vi "RemoveControl.vi"(7 "Ctrl in":u32, 8 "error in":errorcluster, 9 "delay in":u32, 10 "Attrs array in":T1[](array[typedef]), 11 "Ctrl array in":u32[](array[numeric])) -> (0 "error out":errorcluster, 1 "delay out":u32, 2 "Attrs array out":T1[](array[typedef]), 3 "Ctrl array out":u32[](array[numeric]), 4 "stop?":bool)   [LabVIEW 2012, in "Spinner.xctl"]
uses:
  Spinner.xctl
  Attrs.ctl
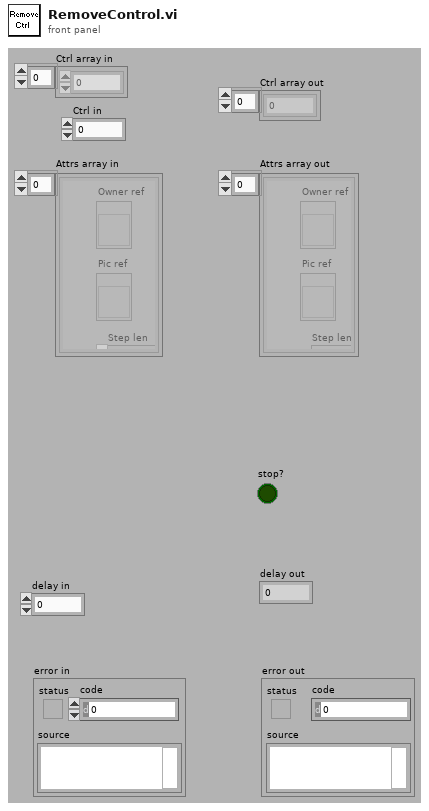
[diagram p1: front panel]
types:
  T1 = typedef "Spinner.xctl/Attrs.ctl" = cluster{"Owner ref":refnum<vi>, "Pic ref":refnum<vi>, "Step len":dbl, "Imgs":picture[], "Current phase":dbl}
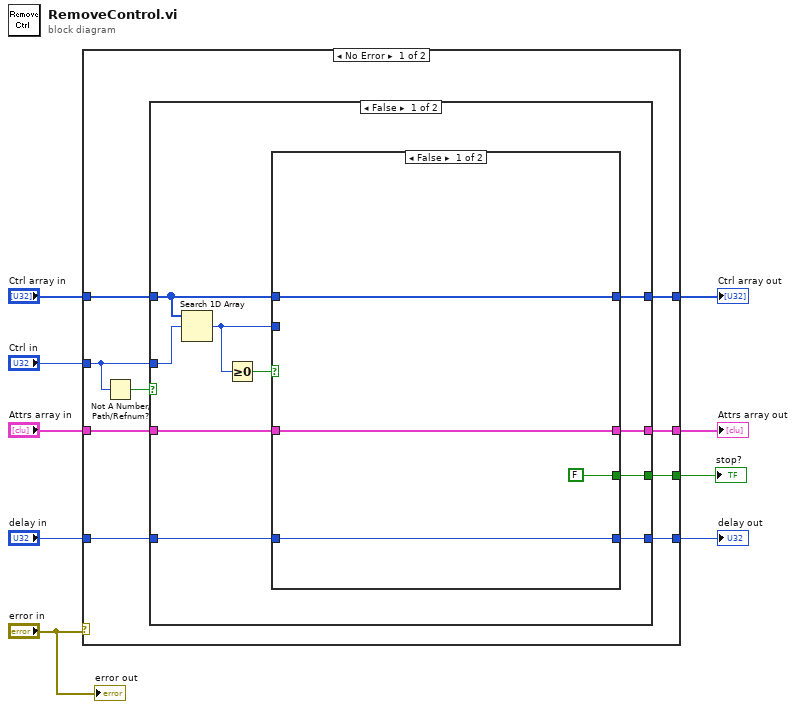
[diagram p0: block diagram]
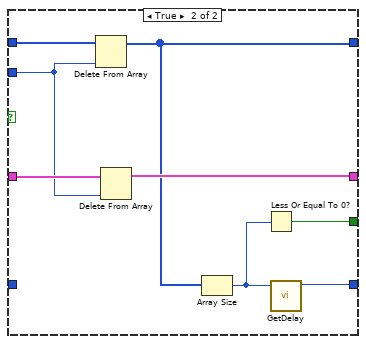
[diagram p2: hidden frame]
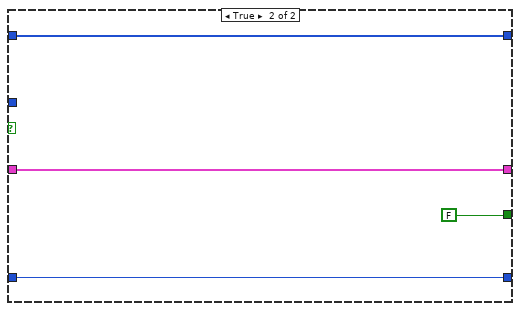
[diagram p3: hidden frame]
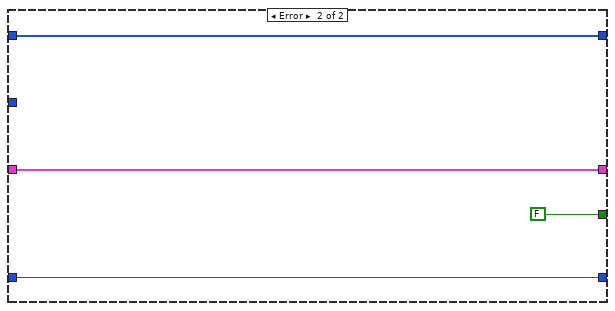
[diagram p4: hidden frame]
diagram:
  n1 = case shown="No Error" "error in" {
    tunnel: "Ctrl in" -> [w16 _]
    tunnel: "Ctrl array in" -> [w17 w48]
    tunnel: "Attrs array in" -> [w15 w47]
    tunnel: [w14 w47] -> w6
    tunnel: [w13 w48] -> w5
    tunnel: [w12 w46] -> w4
    tunnel: "delay in" -> [w11 w46]
    tunnel: [w10 FALSE] -> w1
    frame No Error {
      n2 = Not A Number/Path/Refnum?(number/path/refnum=w16) -> (NaN/Path/Refnum?=w18:bool)
      n3 = case shown="False" w18 {
        tunnel: w17 -> [w25 w44]
        tunnel: w16 -> [w24 _]
        tunnel: w15 -> [w27 w43]
        tunnel: [w26 w43] -> w14
        tunnel: [w23 w44] -> w13
        tunnel: [w22 w42] -> w12
        tunnel: w11 -> [w21 w42]
        tunnel: [w19 FALSE] -> w10
        frame False {
          n4 = Search 1D Array(1D array=w25, element=w24) -> (index of element=w20:i32)  [unwired: 1 in]
          n5 = Greater Or Equal To 0?(x=w20) -> (x >= 0?=w28:bool)
          n6 = case shown="False" w28 {
            tunnel: w27 -> [w31 w39]
            tunnel: [w31 w37] -> w26
            tunnel: w25 -> [w32 w40]
            tunnel: [w32 w35] -> w23
            tunnel: [w30 w36] -> w22
            tunnel: w21 -> [w30 _]
            tunnel: w20 -> [_ w38]
            tunnel: [FALSE w33] -> w19
            frame False {
            }
            frame True {
              n7 = Delete From Array(array=w40, index=w38) -> (array with subset deleted=w35:u32[])  [unwired: 1 in, 1 out]
              n8 = Delete From Array(array=w39, index=w38) -> (array with subset deleted=w37:T1[])  [unwired: 1 in, 1 out]
              n9 = Array Size(array=w35) -> (size(s)=w34:i32)
              n10 = Less Or Equal To 0?(x=w34) -> (x <= 0?=w33:bool)
              n11 = call "GetDelay.vi"("Count"=w34) -> ("Delay"=w36:u32)  [unwired: 9 in, 1 out]
            }
          }
        }
        frame True {
        }
      }
    }
    frame Error {
    }
  }
  "Attrs array out" <- w6
  "Ctrl array out" <- w5
  "delay out" <- w4
  "stop?" <- w1
  "error out" <- "error in"
